vi "Fit.vi"(8 "error in (no error)":errorcluster caption="entrée d'erreur (pas d'erreur)", 10 "Image":string[][](array[string]), 11 "PatchExtractor.lvclass":refnum<class "PatchExtractor.lvclass">) -> (0 "error out":errorcluster caption="sortie d'erreur", 2 "String Data":string, 3 "PatchExtractor.lvclass":refnum<class "PatchExtractor.lvclass">)   [LabVIEW 2020, in "PatchExtractor.lvclass"]
doc: "Do nothing and return the estimator unchanged.\n\nThis method is just there to implement the usual API and hence work in pipelines.\n\nReturns :\n\n- String : OK"
uses:
  PatchExtractor.lvclass
  PatchExtractor.lvclass/PatchExtractor.ctl
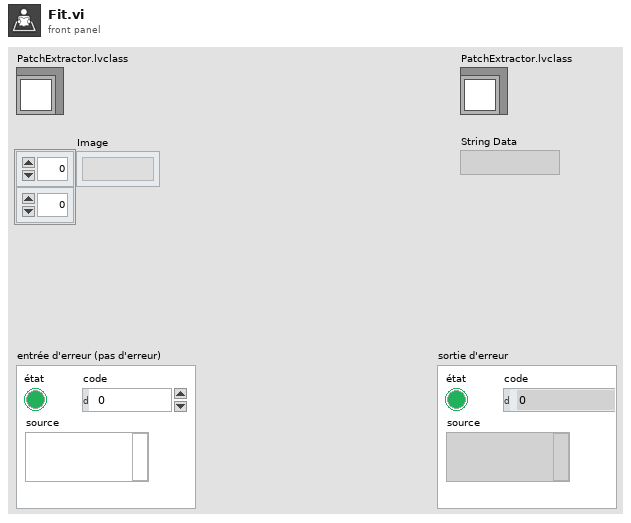
[diagram p1: front panel]
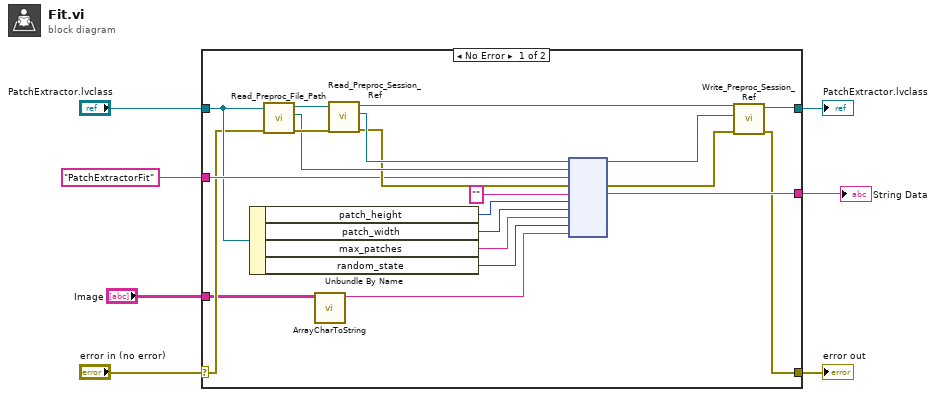
[diagram p0: block diagram]
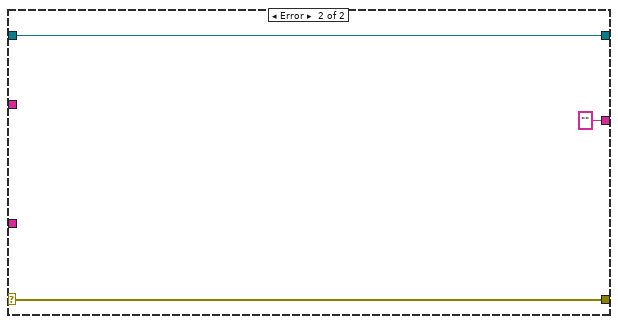
[diagram p2: hidden frame]
diagram:
  n1 = case shown="No Error" "error in (no error)" {
    selector: "error in (no error)" -> [w10 w31]
    tunnel: [w11 w31] -> w6
    tunnel: [w12 w30] -> w4
    tunnel: "PatchExtractor.lvclass" -> [w17 w30]
    tunnel: "PatchExtractorFit" ("Fonction") -> [w19 _]
    tunnel: [w18 ""] -> w2
    tunnel: "Image" -> [w9 _]
    frame No Error {
      n2 = Unbundle By Name(w17) -> ("patch_height"=w16:i32, "patch_width"=w15:i32, "max_patches"=w14:string, "random_state"=w13:i32)
      n3 = call-dynamic "Read_Preproc_File_Path.vi"("error in (no error)"=w10, "Python in"=w17) -> ("error out"=w27:errorcluster, "File_Path"=w26:path, "Python out"=w28:refnum<class "PatchExtractor.lvclass">)  [unwired: 7 in]
      n4 = call "ArrayCharToString.vi"("TAB"=w9) -> ("Instruction"=w8:string)  [unwired: 10 in]
      n5 = call-dynamic "Read_Preproc_Session_Ref.vi"("error in (no error)"=w27, "Python in"=w28) -> ("error out"=w24:errorcluster, "Session_ref"=w25:refnum<k35>, "Python out"=w23:refnum<class "PatchExtractor.lvclass">)  [unwired: 7 in]
      n6 = node(w25, w26, w19, w24, "", w16, w15, w14, w13, w8) -> (w21:refnum<k35>, w22:errorcluster, w18:string)  [unwired: 5 in, 2 out]
      n7 = call-dynamic "Write_Preproc_Session_Ref.vi"("error in (no error)"=w22, "Session_ref"=w21, "Python in"=w23) -> ("error out"=w11:errorcluster, "Python out"=w12:refnum<class "PatchExtractor.lvclass">)  [unwired: 7 in]
    }
    frame Error {
    }
  }
  "error out" <- w6
  "PatchExtractor.lvclass" <- w4
  "String Data" <- w2
